vi "PH_Sixpack_Switch.PC _Information.vi"(0 "i ref in":refnum<vi>, 2 "Axis Information":T1, 5 "error IO":errorcluster) -> (14 "i ref out":refnum<vi>, 19 "error out":errorcluster)   [LabVIEW 2014, in "PH_Sixpack_Switch.lvlib"]
doc: "This VI stores data in on attributes and sets GUI elements."
uses:
  PH_Sixpack_Switch.lvlib
  PH_Basics/PH_Stepmotor_BaseClass/PH_Stepmotor_BaseClass.Axis Information.ctl
  PH_Basics/PH_Stepmotor_BaseClass/PH_Stepmotor_BaseClass.Axis Activity.ctl
  PH_Basics/PH_StatusHandler/PH_StatusHandler.Status.ctl
  PH_Basics/PH_Stepmotor_BaseClass/PH_Stepmotor_BaseClass.Axis Direction.ctl
  PH_Basics/PH_Stepmotor_BaseClass/PH_Stepmotor_BaseClass.lvlib
  PH_Basics/PH_StatusHandler/PH_StatusHandler.lvlib
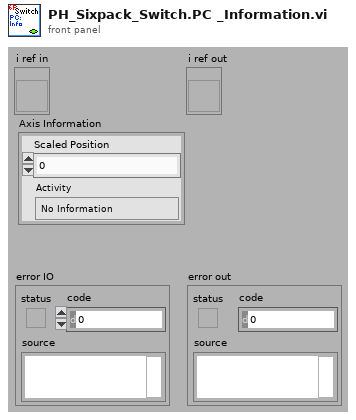
[diagram p1: front panel]
types:
  T1 = typedef "PH_Stepmotor_BaseClass.lvlib/PH_Stepmotor_BaseClass.Axis Information.ctl" = cluster{"Scaled Position":dbl, "Activity":T2}
  T2 = typedef "PH_Stepmotor_BaseClass.lvlib/PH_Stepmotor_BaseClass.Axis Activity.ctl" = enum16{"No Information", "stopped", "running", "Failure", "Alarm", "stopped at backward ES", "stopped at foreward ES"}
  T3 = typedef "PH_StatusHandler.lvlib/PH_StatusHandler.Status.ctl" = i16
  T4 = typedef "PH_Stepmotor_BaseClass.lvlib/PH_Stepmotor_BaseClass.Axis Direction.ctl" = enum16{"forward", "backward"}
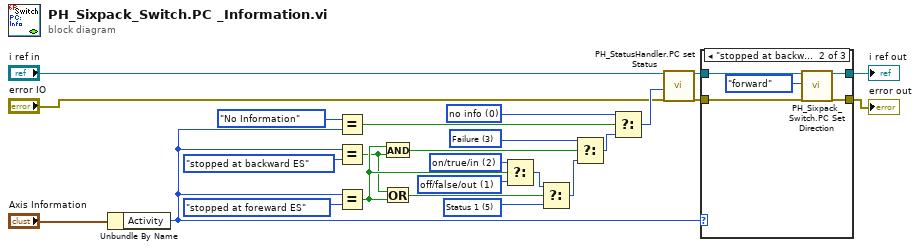
[diagram p0: block diagram]
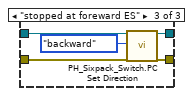
[diagram p3: hidden frame]
diagram:
  w15 = T3 2 items=["no info", "off/false/out", "on/true/in", "Failure", "Alarm", "Status 1", "Status 2", "Status 3"] ("t")
  w16 = T3 1 items=["no info", "off/false/out", "on/true/in", "Failure", "Alarm", "Status 1", "Status 2", "Status 3"] ("t")
  w19 = T3 5 items=["no info", "off/false/out", "on/true/in", "Failure", "Alarm", "Status 1", "Status 2", "Status 3"] ("t")
  w21 = T3 3 items=["no info", "off/false/out", "on/true/in", "Failure", "Alarm", "Status 1", "Status 2", "Status 3"] ("t")
  w7 = T3 0 items=["no info", "off/false/out", "on/true/in", "Failure", "Alarm", "Status 1", "Status 2", "Status 3"] ("Status")
  n1 = Unbundle By Name("Axis Information") -> ("Activity"=w5:T2)
  n2 = Equal?(x=PH_Stepmotor_BaseClass.Axis_Activity."No Information", y=w5) -> (x = y?=w8:bool)
  n3 = Equal?(x=w5, y=PH_Stepmotor_BaseClass.Axis_Activity."stopped at backward ES") -> (x = y?=w11:bool)
  n4 = Equal?(x=w5, y=PH_Stepmotor_BaseClass.Axis_Activity."stopped at foreward ES") -> (x = y?=w17:bool)
  n5 = And(x=w17, y=w11) -> (x .and. y?=w22:bool)
  n6 = Or(x=w11, y=w17) -> (x .or. y?=w20:bool)
  n7 = Select(t=w15, s=w17, f=w16) -> (s? t:f=w14:T3)
  n8 = Select(t=w14, s=w20, f=w19) -> (s? t:f=w18:T3)
  n9 = Select(t=w21, s=w22, f=w18) -> (s? t:f=w6:T3)
  n10 = Select(t=w7, s=w8, f=w6) -> (s? t:f=w13:T3)
  n11 = call "PH_StatusHandler.PC set Status.vi"("i ref in"="i ref in", "Status"=w13, "error in (no error)"="error IO") -> ("i ref out"=w4:refnum<vi>, "error out"=w3:errorcluster)  [unwired: 15 in]
  n12 = case shown="\"stopped at backward ES\"" w5 {
    tunnel: [w27 w32 w37] -> w25
    tunnel: w4 -> [w27 w31 w36]
    tunnel: [w26 w30 w35] -> w24
    tunnel: w3 -> [w26 w29 w34]
    frame Default {
    }
    frame "stopped at backward ES" {
      n13 = call "PH_Sixpack_Switch.PC Set Direction.vi"("i ref in"=w31, "Direction"=PH_Stepmotor_BaseClass.Axis_Direction."forward", "error IO"=w29) -> ("i ref out"=w32:refnum<vi>, "error out"=w30:errorcluster)  [unwired: 15 in]
    }
    frame "stopped at foreward ES" {
      n14 = call "PH_Sixpack_Switch.PC Set Direction.vi"("i ref in"=w36, "Direction"=PH_Stepmotor_BaseClass.Axis_Direction."backward", "error IO"=w34) -> ("i ref out"=w37:refnum<vi>, "error out"=w35:errorcluster)  [unwired: 15 in]
    }
  }
  "error out" <- w24
  "i ref out" <- w25
